vi "FlpLib InductorVtoI 1.vi"(1 "L":sgl, 2 "dT":sgl, 5 "Vpos":sgl, 7 "Vneg":sgl, 12 "inital current":sgl) -> (8 "Current":sgl)   [LabVIEW 2017]
uses:
  <userlib>/_NI FLP Library/FPGA/outsideSCTL/FlpLib Subtract Shared Instance 1.vi
  Calculus/Integrator/FlpLib Integrator 1.vi
  <userlib>/_NI FLP Library/FPGA/outsideSCTL/FlpLib Divide Shared Instance 1.vi
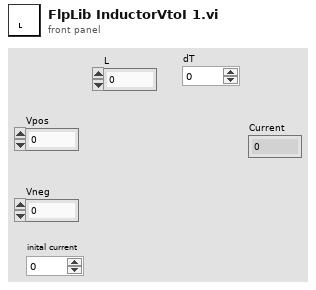
[diagram p1: front panel]
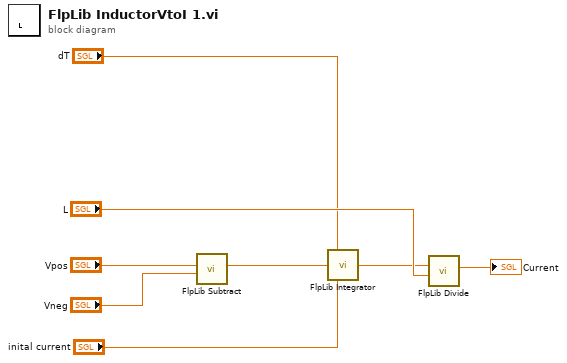
[diagram p0: block diagram]
diagram:
  n1 = call-poly <userlib>:"FlpLib Subtract.vi"("y"="Vneg", "x"="Vpos") -> ("x-y"=w4:sgl)  [unwired: 5 in]
  n2 = call-poly "FlpLib Integrator.vi"("dt"="dT", "dx"=w4, "initial"="inital current") -> ("x"=w2:sgl)  [unwired: 12 in]
  n3 = call-poly <userlib>:"FlpLib Divide.vi"("y"="L", "x"=w2) -> ("x/y"=→"Current":sgl)  [unwired: 5 in]
